vi "NiXnet WriteSignalWaveform.vi"(6 "contextId":T1, 8 "error in":errorcluster, 9 "timeout (ms)":i32=-1, 10 "Request Data":T3, 11 "gRPC ID":T1) -> (0 "error out":errorcluster, 2 "Response Data":T2, 3 "gRPC ID out":T1)   [LabVIEW 2025, in "grpc-xnet_client.lvlib"]
uses:
  grpc-xnet_client.lvlib
  <vilib>/gRPC/LabVIEW gRPC Library/Shared/grpcId.ctl
  RPC Messages/nixnet_grpc_WriteSignalWaveformRequest.ctl
  RPC Messages/nixnet_grpc_WriteSignalWaveformRequest_timeout_enum/nixnet_grpc_WriteSignalWaveformRequest_timeout_enum.lvclass
  RPC Messages/nidevice_grpc_Session.ctl
  RPC Messages/nixnet_grpc_WriteSignalWaveformResponse.ctl
  RPC Messages/nixnet_grpc_WriteSignalWaveformResponse_Flat.ctl
  RPC Messages/nixnet_grpc_WriteSignalWaveformRequest_timeout_enum/nixnet_grpc_WriteSignalWaveformRequest_timeout_enum.lvclass/nixnet_grpc_WriteSignalWaveformRequest_timeout_enum.ctl
  14035477-4c25-4107-8ed5-d0c4ef420ce5.vi
  RPC Messages/RichToFlatnidevice_grpc_Session.vi
  RPC Messages/nixnet_grpc_WriteSignalWaveformRequest_timeout_enum/GetActiveFieldIndex.vi
  RPC Messages/nixnet_grpc_WriteSignalWaveformRequest_timeout_enum/Gettimeout.vi
  RPC Messages/nixnet_grpc_WriteSignalWaveformRequest_timeout_enum/Gettimeout_raw.vi
  <vilib>/gRPC/LabVIEW gRPC Library/Shared/TranslateGrpcError.vi
  <vilib>/gRPC/LabVIEW gRPC Library/Shared/Wait On Occurrence.vi
  <vilib>/gRPC/LabVIEW gRPC Library/Shared/Is Feature Enabled.vi
  <vilib>/gRPC/LabVIEW gRPC Library/Server API/Server/Get Server DLL Path.vi
  <vilib>/Utility/error.llb/Error Cluster From Error Code.vi
  <vilib>/gRPC/LabVIEW gRPC Library/grpc-lvsupport-release.lvlib
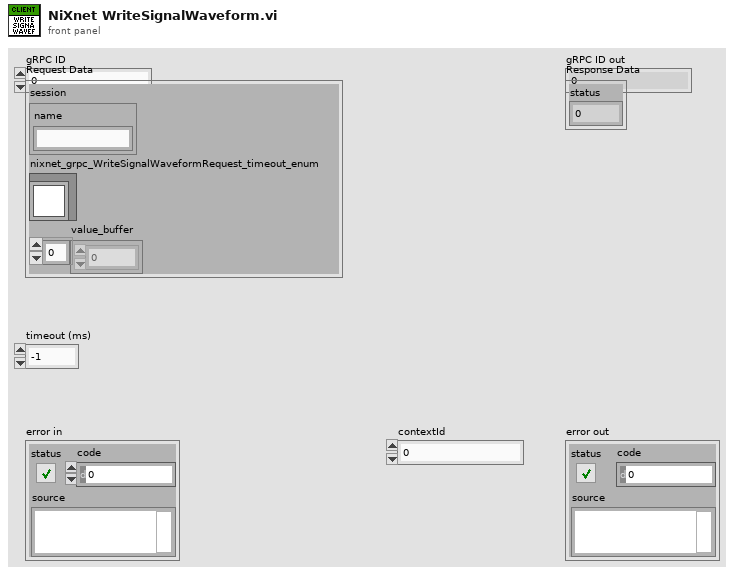
[diagram p1: front panel]
types:
  T1 = typedef "grpc-lvsupport-release.lvlib/grpcId.ctl" = u64
  T2 = typedef "grpc-xnet_client.lvlib/nixnet_grpc_WriteSignalWaveformResponse.ctl" = cluster{"status":i32}
  T3 = typedef "grpc-xnet_client.lvlib/nixnet_grpc_WriteSignalWaveformRequest.ctl" = cluster{"session":T4, "nixnet_grpc_WriteSignalWaveformRequest_timeout_enum":refnum<class "nixnet_grpc_WriteSignalWaveformRequest_timeout_enum.lvclass">, "value_buffer":dbl[]}
  T4 = typedef "grpc-xnet_client.lvlib/nidevice_grpc_Session.ctl" = cluster{"name":string}
  T5 = typedef "grpc-xnet_client.lvlib/nixnet_grpc_WriteSignalWaveformResponse_Flat.ctl" = cluster{"status":i32}
  T6 = typedef "grpc-xnet_client.lvlib/nixnet_grpc_WriteSignalWaveformRequest_Flat.ctl" = cluster{"session":T7, "nixnet_grpc_WriteSignalWaveformRequest_timeout_enum_selected_index":i32, "timeout":T8, "timeout_raw":dbl, "value_buffer":dbl[]}
  T7 = typedef "grpc-xnet_client.lvlib/nidevice_grpc_Session_Flat.ctl" = cluster{"name":string}
  T8 = typedef "grpc-xnet_client.lvlib/nixnet_grpc_TimeOut.ctl" = enum32{"TIME_OUT_NONE", "TIME_OUT_INFINITE"}
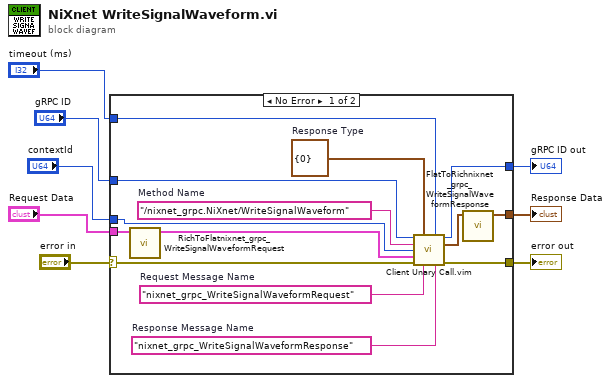
[diagram p0: block diagram]
diagram:
  n1 = case shown="No Error" "error in" {
    selector: "error in" -> [w18 w23]
    tunnel: [w17 w23] -> w7
    tunnel: "gRPC ID" -> [w16 w24]
    tunnel: [w15 w24] -> w5
    tunnel: "Request Data" -> [w12 _]
    tunnel: [w9 _] -> w3
    tunnel: "timeout (ms)" -> [w14 _]
    tunnel: "contextId" -> [w13 _]
    frame No Error {
      w19 = "nixnet_grpc_WriteSignalWaveformResponse"  # Response Message Name
      w20 = "nixnet_grpc_WriteSignalWaveformRequest"  # Request Message Name
      w21 = T5 {"status"=0}  # Response Type
      w22 = "/nixnet_grpc.NiXnet/WriteSignalWaveform"  # Method Name
      n2 = call "RichToFlatnixnet_grpc_WriteSignalWaveformRequest.vi"("InputCluster"=w12) -> ("OutputCluster"=w11:T6)  [unwired: 10 in]
      n3 = call "Client Unary Call.vim"("ClientID in"=w16, "Response Type"=w21, "timeout (ms)"=w14, "Method Name"=w22, "contextId"=w13, "Request Data"=w11, "error in"=w18, "Request Message Name"=w20, "Response Message Name"=w19) -> ("ClientID out"=w15:u64, "Response Data"=w10:T5, "error out"=w17:errorcluster)  [unwired: 4 in]
      n4 = call "FlatToRichnixnet_grpc_WriteSignalWaveformResponse.vi"("InputCluster"=w10) -> ("OutputCluster"=w9:T2)  [unwired: 10 in]
    }
    frame Error {
    }
  }
  "error out" <- w7
  "gRPC ID out" <- w5
  "Response Data" <- w3
